vi "square_roi.vi"(8 "Error In":errorcluster, 10 "ROI Size":T1, 11 "ROI In":T2) -> (0 "Error Out":errorcluster, 3 "ROI Out":T2)   [LabVIEW 2019]
doc: "Takes a ROI and if it's a point, makes it a square around that point. If it's not a point, then it just passes the ROI on through."
uses:
  sections_roi_size_enum_typedef.ctl
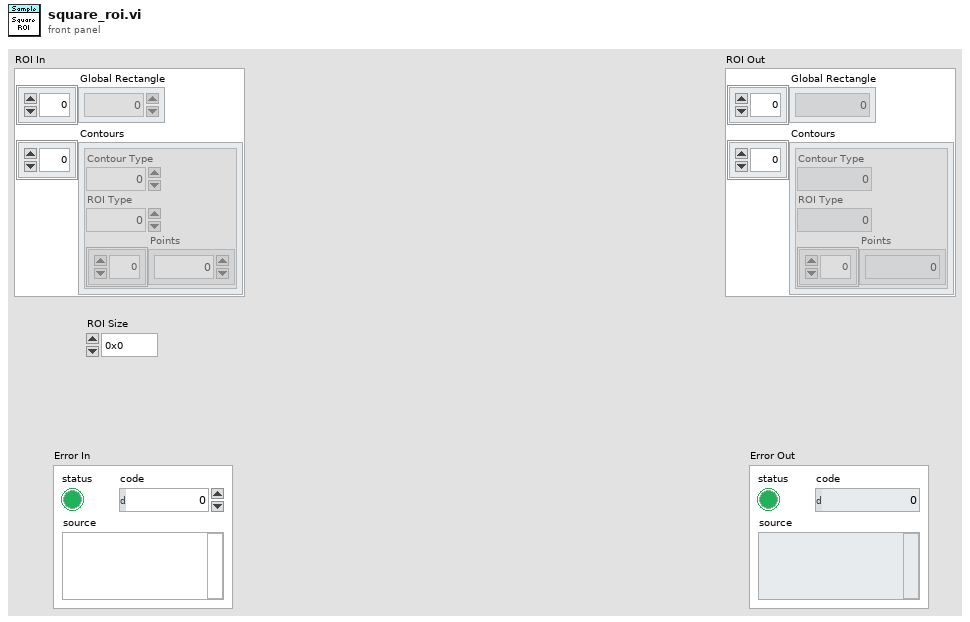
[diagram p1: front panel]
types:
  T1 = typedef "sections_roi_size_enum_typedef.ctl" = enum16{"0x0", "1x1", "2x2", "3x3", "4x4", "5x5", "6x6"}
  T2 = cluster{"Global Rectangle":i32[], "Contours":cluster{"Contour Type":u32, "ROI Type":u32, "Points":i32[]}[]}
  T3 = cluster{"Contour Type":u32, "ROI Type":u32, "Points":i32[]}[]
  T4 = cluster{"Contour Type":u32, "ROI Type":u32, "Points":i32[]}
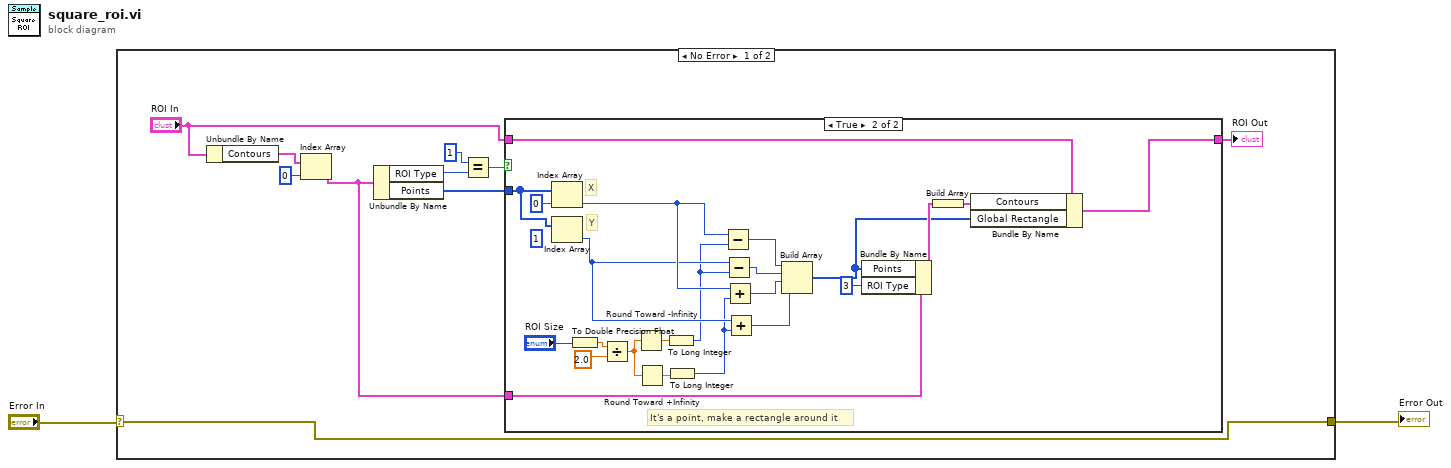
[diagram p0: block diagram]
diagram:
  n1 = case shown="No Error" "Error In" {
    selector: "Error In" -> [w3 w37]
    tunnel: [w3 w37] -> w1
    frame No Error {
      n2 = Unbundle By Name("ROI In") -> ("Contours"=w12:T3)
      n3 = Index Array(array=w12, index=0) -> (element=w6:T4)
      n4 = Unbundle By Name(w6) -> ("ROI Type"=w10:u32, "Points"=w7:i32[])
      n5 = Equal?(x=u32 1, y=w10) -> (x = y?=w8:bool)
      n6 = case shown="True" w8 {
        tunnel: w7 -> [_ w29]
        tunnel: w6 -> [_ w20]
        tunnel: "ROI In" -> [w13 w18]
        tunnel: [w13 w14] -> w4
        frame False {
          # "Not a point, just pass through"
        }
        frame True {
          (unwired) 1 ("index")
          # "Y"
          # "X"
          # "It's a point, make a rectangle around it"
          n7 = Index Array(array=w29, index=0) -> (element=w28:i32)
          n8 = Index Array(array=w29) -> (element=w27:i32)  [unwired: 1 in]
          n9 = To Double Precision Float(number="ROI Size") -> (double precision float=w35:dbl)
          n10 = Divide(x=w35, y=2.0) -> (x/y=w33:dbl)
          n11 = Round Toward -Infinity(1:w33) -> (0:w32:dbl)
          n12 = Round Toward +Infinity(x=w33) -> (ceil(x): smallest int >= x=w31:dbl)
          n13 = To Long Integer(number=w32) -> (32bit integer=w26:i32)
          n14 = To Long Integer(number=w31) -> (32bit integer=w25:i32)
          n15 = Subtract(x=w28, y=w26) -> (x-y=w24:i32)
          n16 = Subtract(x=w27, y=w26) -> (x-y=w23:i32)
          n17 = Add(x=w28, y=w25) -> (x+y=w22:i32)
          n18 = Add(x=w27, y=w25) -> (x+y=w21:i32)
          n19 = Build Array(w24, w23, w22, w21) -> (w15:i32[])
          n20 = Bundle By Name(cluster=w20, "Points"=w15, "ROI Type"=u32 3) -> (w16:T4)
          n21 = Build Array(w16) -> (w17:T3)
          n22 = Bundle By Name(cluster=w18, "Contours"=w17, "Global Rectangle"=w15) -> (w14:T2)
        }
      }
      "ROI Out" <- w4
    }
    frame Error {
    }
  }
  "Error Out" <- w1
